vi "I-SRC Shutdown (26XX).vi"(8 "error in (no error)":errorcluster, 11 "VISA resource name in":refnum<visa-resource-name>) -> (0 "error out":errorcluster, 3 "VISA resource name out":refnum<visa-resource-name>)   [LabVIEW 2016, in "Hall Effect Library.lvlib"]
uses:
  Hall Effect Library.lvlib
  <instrlib>/ke26xx/ke26xx.lvlib
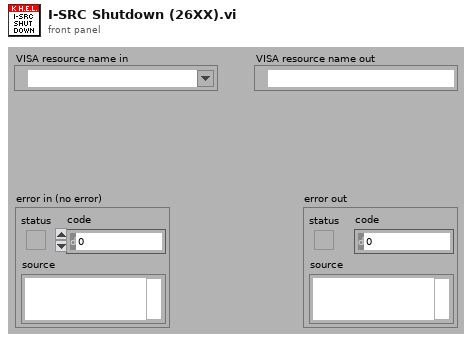
[diagram p1: front panel]
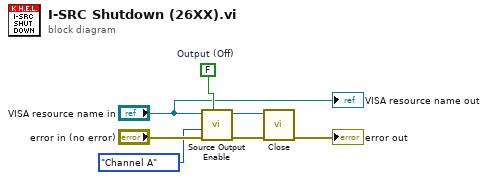
[diagram p0: block diagram]
diagram:
  w3 = FALSE  # Output (Off)
  n1 = call <instrlib>:"Source Output Enable.vi"("Output (Off)"=w3, "error in (no error)"="error in (no error)", "Channel (Channel A)"=enum32{"Channel A", "Channel B"}."Channel A", "VISA resource name"="VISA resource name in") -> ("error out"=w7:errorcluster, "VISA resource name out"=w6:refnum<visa-resource-name>)  [unwired: 1 in, 5 out]
  n2 = call <instrlib>:"Close.vi"("error in (no error)"=w7, "VISA resource name"=w6) -> ("error out"=→"error out":errorcluster)  [unwired: 9 out]
  "VISA resource name out" <- "VISA resource name in"
